vi "Шифр Хилла.vi"() -> ()   [LabVIEW 2016]
uses:
  <vilib>/Analysis/Matrix/Datatypes/RealMatrix.ctl
  <vilib>/silver_ctls/ArrayMatrixCluster/Real Matrix NI_Silver.ctl
  Dll_Hill/Dll_Hill/Dll_Hill/bin/Debug/Dll_Hill.dll
  <vilib>/Analysis/baseanly.llb/Real Determinant.vi
  <vilib>/Analysis/baseanly.llb/Vector x A.vi
  <vilib>/Analysis/baseanly.llb/Real A x B.vi
  <vilib>/Analysis/Matrix/Numeric/Conversions/Array To Matrix - RA.vi
  <vilib>/Analysis/Matrix/Numeric/Conversions/Matrix To Array - RM.vi
  <vilib>/Analysis/NI_AALBase.lvlib
  <vilib>/Analysis/Matrix/NI_Matrix.lvlib
panel:
  in  "Главное меню":T1(tab)
  in  "Укажите путь к входному алфавиту":path
  in  "Путь к алфавиту":bool
  in  "Выход":bool
  out "Входной алфавит":string
  out "index":i32[](array[numeric])
  in  "Введите входное слово":string
  in  "Введите ключ":string
  in  "Получение ключа и входного сообщения":bool
  out "Полученный ключ":string
  out "Матрица ключа":T2
  in  "Строки матрицы ключа":i32
  in  "Столбцы матрицы ключа":i32
  out "Полученное входное слово":string
  out "Вектор входного слова":i32[](array[numeric])
  in  "дл.исх.сообщ.":i32
  out "Зашифрованный вектор_2":string[][](table)
  in  "Шифрование":bool
  out "Матрица ключа * Матрицу вх. сообщ.":dbl[](array[numeric]) format="%.2f"
  out "Зашифрованный вектор":dbl[](array[numeric])
  out "Определитель матрицы ключа":i32
  in  "Пользовательский пример.\nУкажите путь к файлу  в Подменю\n\"Пользовательский пример\"\nперед нажатием на кнопку - \n\"Пользовательский пример\"":bool
  in  "Расшифрование":bool
  in  "Выход в главное меню":bool
  in  "Подменю":T3(tab)
  out "Зашифрованное сообщение_2":string[][](table)
  in  "Зашифрованное сообщение":string
  in  "Закодированный ключ_р":T4
  in  "Укажите путь к  алфавиту дешифрования":path
  out "Зашифрованный ключ_р_2":string[][](table)
  out "Исходное сообщение":dbl[](array[numeric])
  out "Исходное сообщение":string
  in  "дл.исх.сообщ.":i32
  out "y":i64[](array[numeric])
  out "x":i64[](array[numeric])
  out "d":i64[](array[numeric])
  out "pow":i32
  out "минор":i32
  out "invert_det":i64
  out "опред  минора":T2
  out "Проверка":T2
  out "обратная по модулю к матрице ключа":T2
  out "Матрица миноров":T2
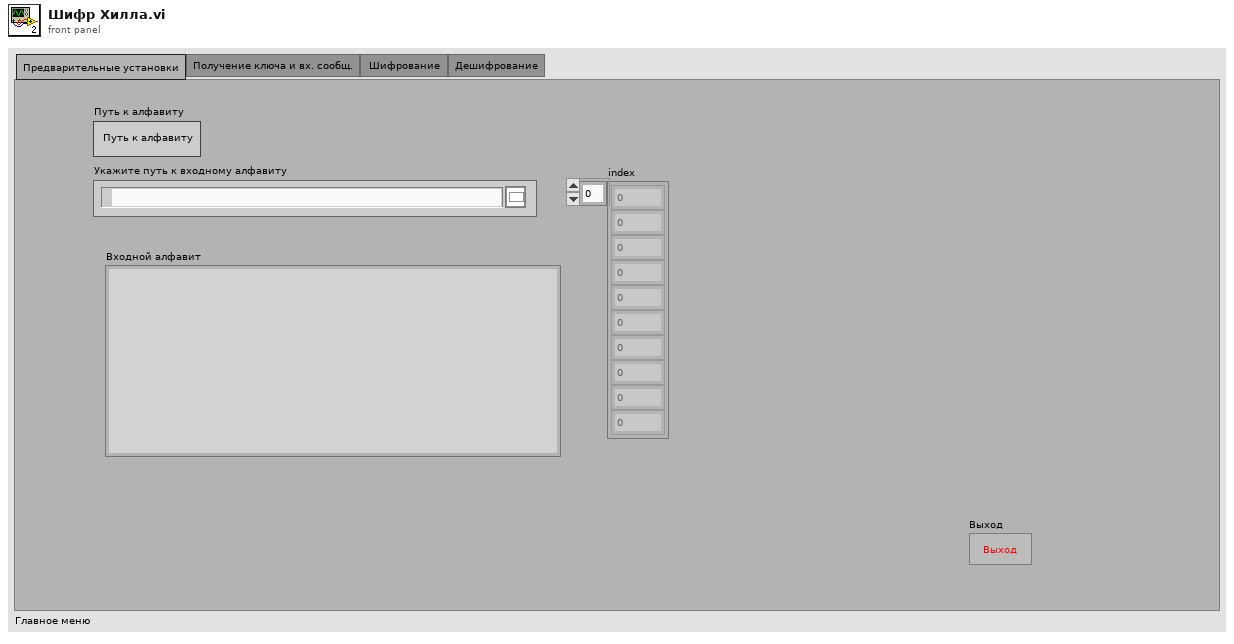
[diagram p1: front panel]
types:
  T1 = enum32{"Предварительные установки", "Получение ключа и вх. сообщ.", "Шифрование ", "Дешифрование"}
  T2 = typedef "NI_Matrix.lvlib/RealMatrix.ctl" = dbl[][]
  T3 = enum32{"Пользовательский пример", "Пользовательский пример шаг_2"}
  T4 = typedef "Real Matrix NI_Silver.ctl" = dbl[][]
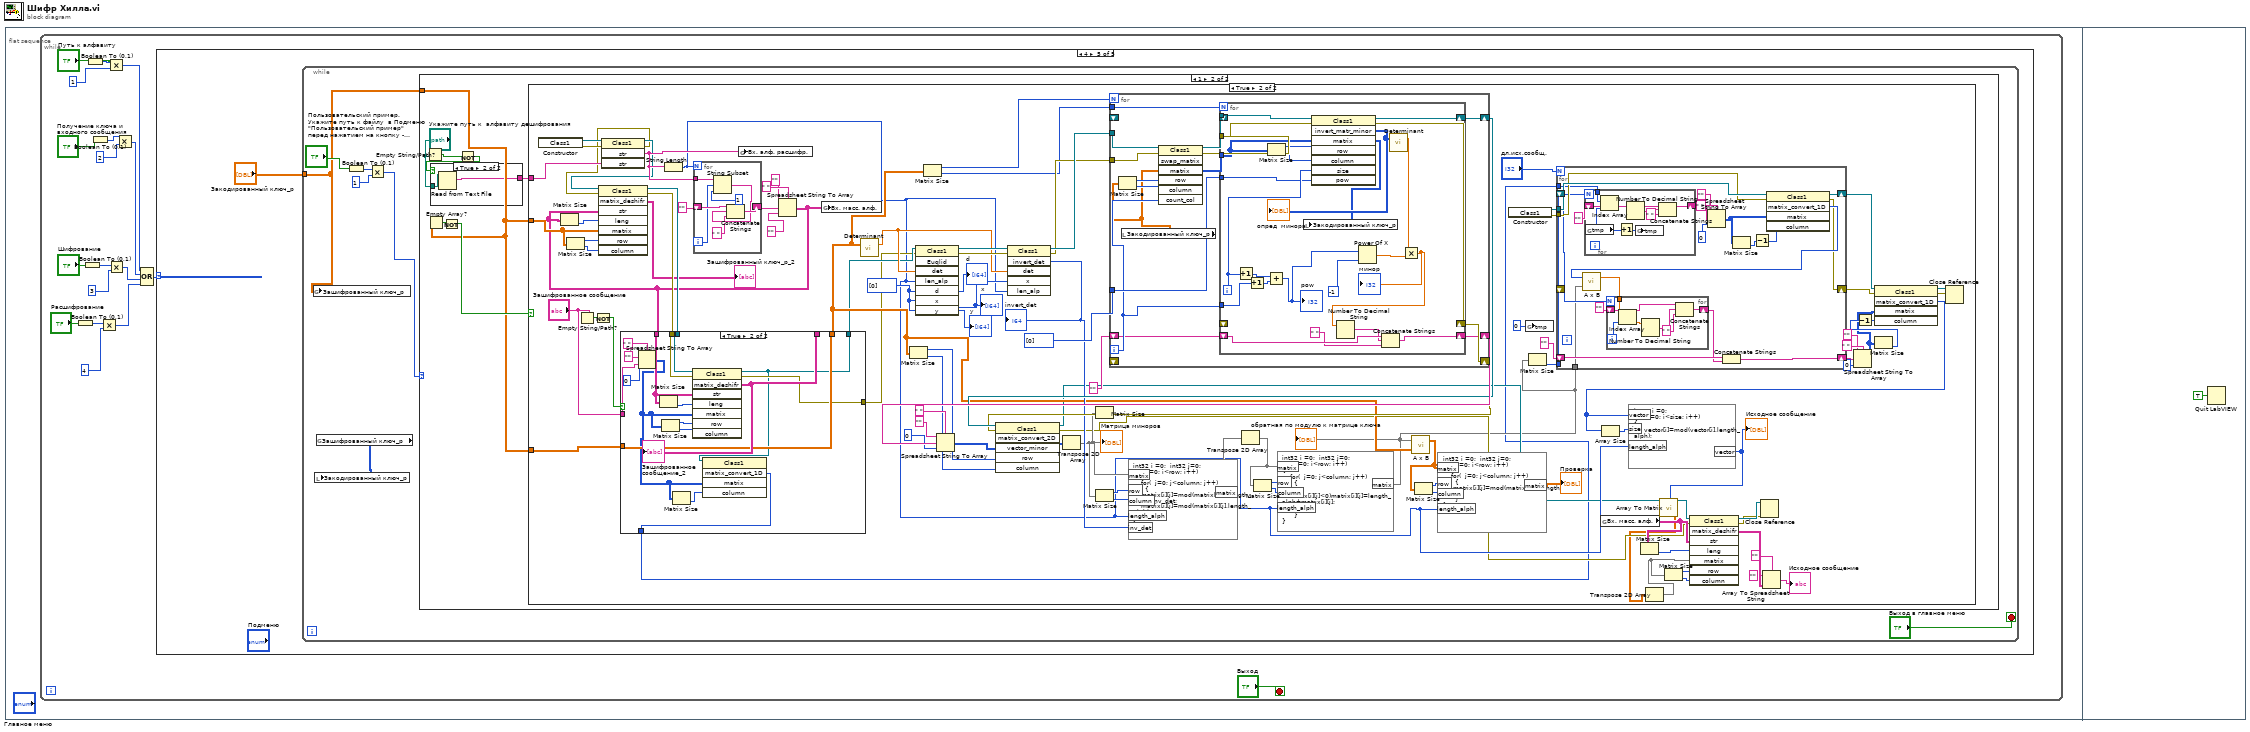
[diagram p0: block diagram]
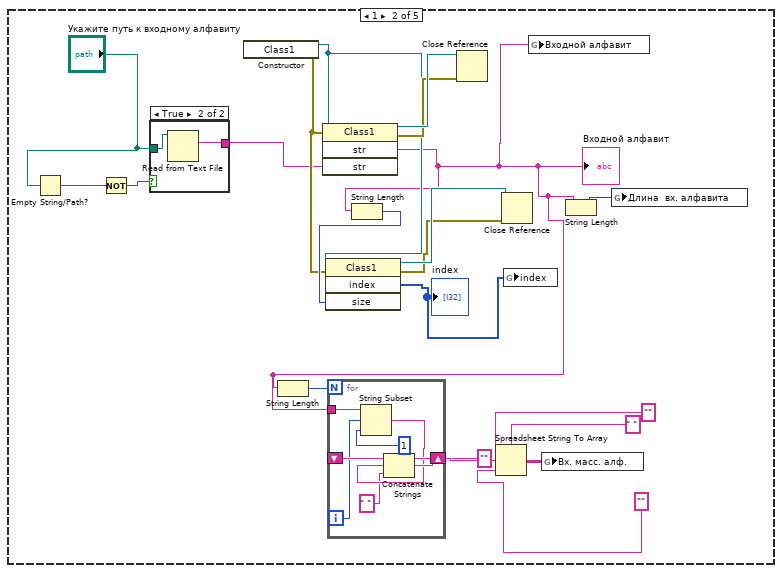
[diagram p3: hidden frame]
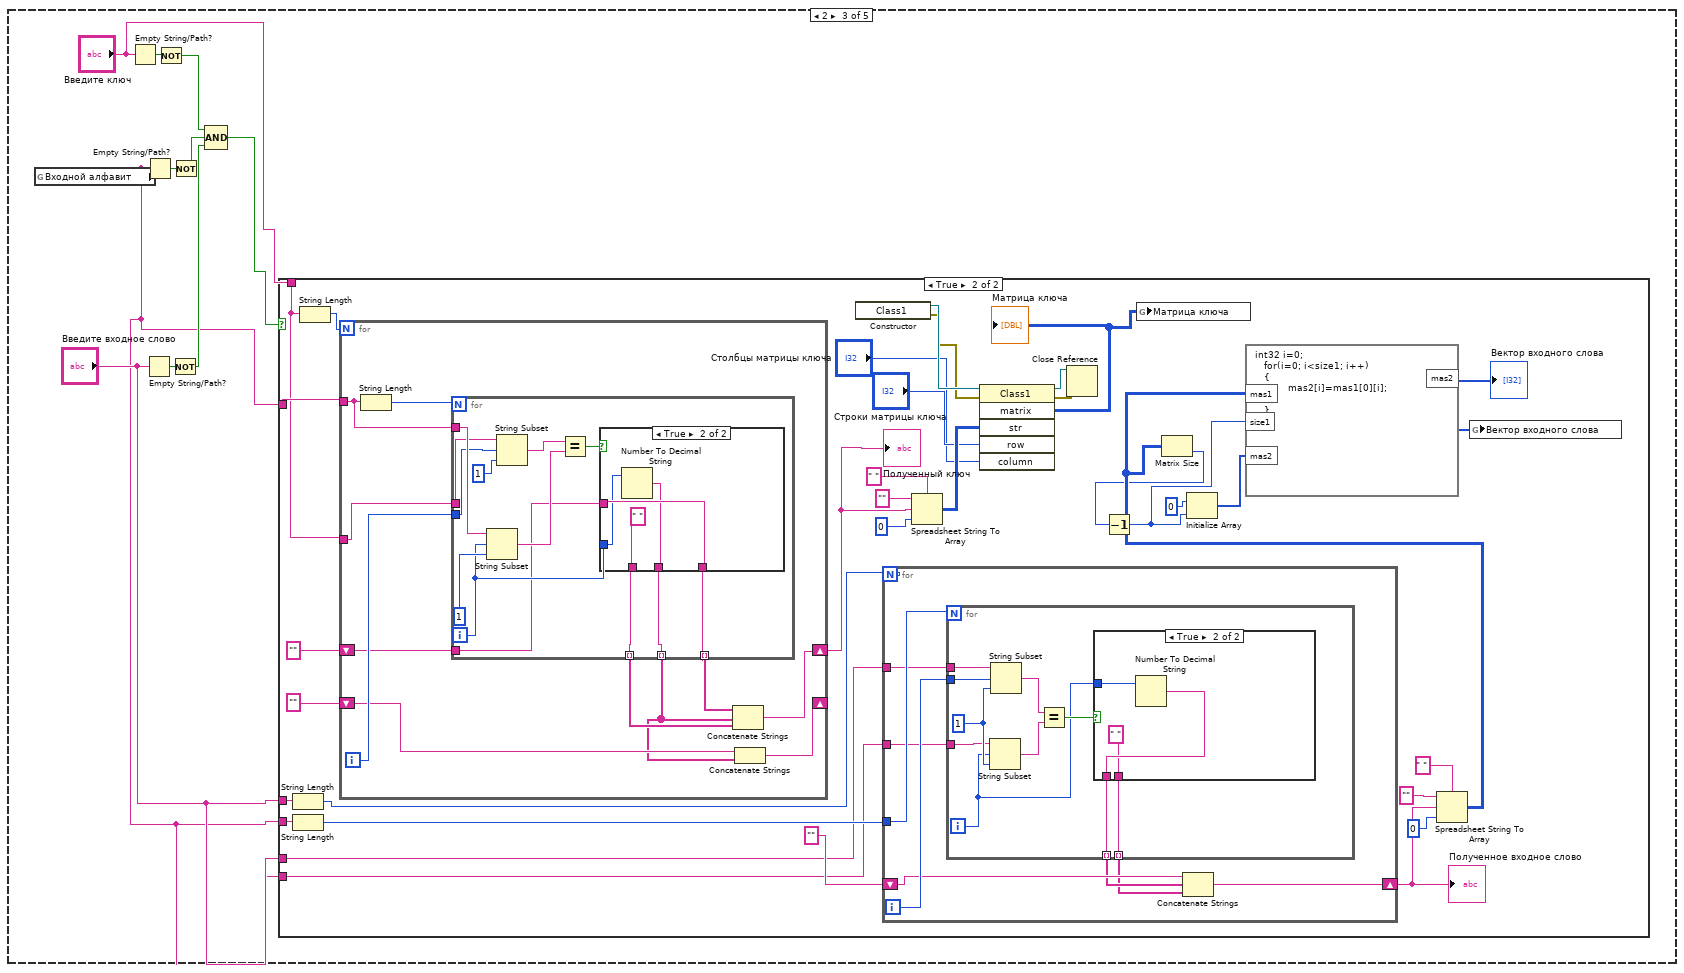
[diagram p5: hidden frame]
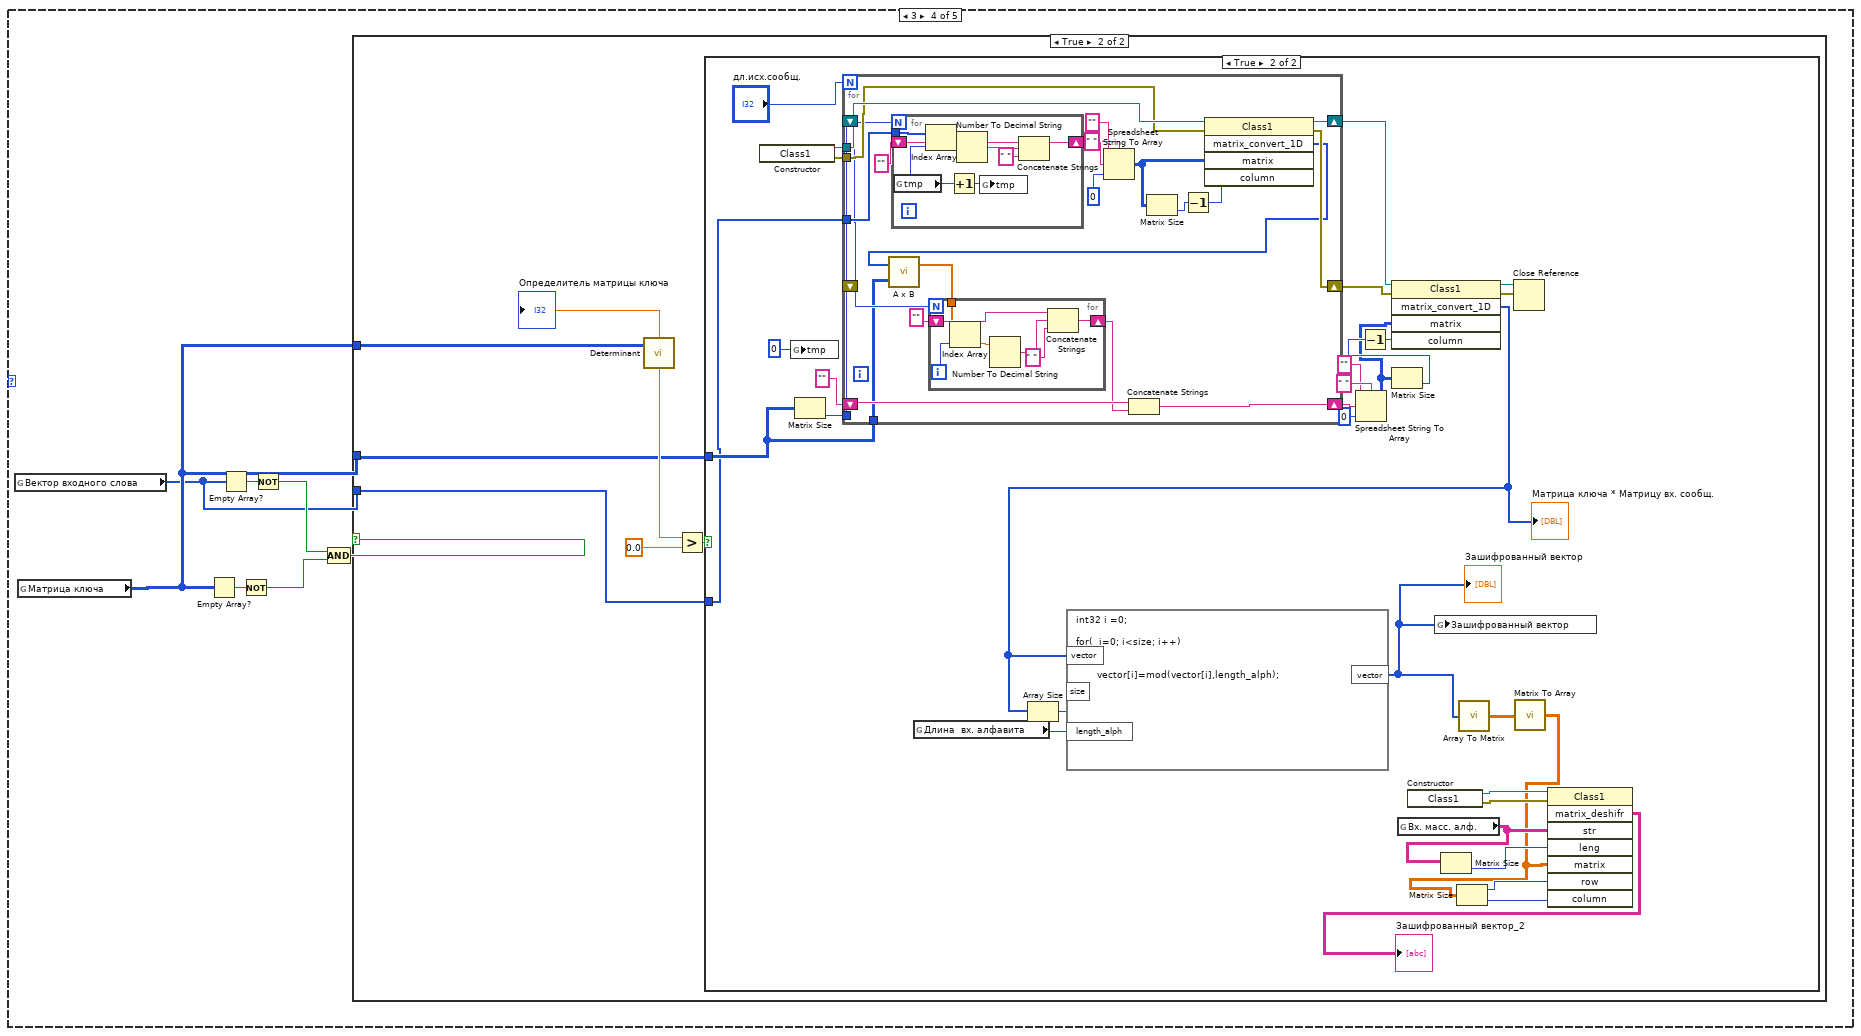
[diagram p9: hidden frame]
diagram:
  n1 = flat-sequence {
    frame #0 {
      n2 = while {
        stop <- "Выход" stop-if-true
        n3 = Boolean To (0,1)(Boolean="Расшифрование") -> (0, 1=w2:i16)
        n4 = Boolean To (0,1)(Boolean="Шифрование") -> (0, 1=w6:i16)
        n5 = Boolean To (0,1)(Boolean="Путь к алфавиту") -> (0, 1=w16:i16)
        n6 = Boolean To (0,1)(Boolean="Получение ключа и входного сообщения") -> (0, 1=w13:i16)
        n7 = Multiply(x=w2, y=4) -> (x*y=w1:i32)
        n8 = Multiply(x=w16, y=1) -> (x*y=w10:i32)
        n9 = Multiply(x=w6, y=3) -> (x*y=w5:i32)
        n10 = Multiply(x=w13, y=2) -> (x*y=w9:i32)
        n11 = Compound Arithmetic op=OR(w10, w9, w5, w1) -> (w15:i32)
        n12 = case shown="4" w15 {
          frame 0, Default {
          }
          frame 1 {
            n13 = Empty String/Path?(string/path="Укажите путь к входному алфавиту") -> (empty?=w31:bool)
            n14 = Not(x=w31) -> (.not. x?=w30:bool)
            n15 = case shown="True" w30 {
              tunnel: "Укажите путь к входному алфавиту" -> [_ w48]
              tunnel: [_ w47] -> w28
              frame False {
              }
              frame True {
                n16 = Read from Text File(file (use dialog)=w48) -> (text=w47:string)  [unwired: 3 in, 3 out]
              }
            }
            n17 = constructor class="Class1"() -> (reference out=w37:refnum<k24>, error out=w35:errorcluster)  [unwired: 3 in, 1 out]
            n18 = invoke class="Class1" method="str"(reference=w37, error in=w35, "str"=w28) -> (reference out=w39:refnum<k24>, error out=w38:errorcluster, "str"=w19:string)  [unwired: 1 in, 1 out]
            "Входной алфавит" <- w19
            n19 = String Length(string=w19) -> (length=w21:i32)
            n20 = for {
              N: w21 -> [_]
              shift-right: [w46] -> w23
              shift-left: "" -> [w45]
              tunnel: w19 -> [w40]
              i -> [w43]
              n21 = String Subset(string=w40, offset (0)=w43, length (rest)=1 ("length (rest)")) -> (substring=w42:string)
              n22 = Concatenate Strings(w45, w42, " ") -> (w46:string)
            }
            n23 = String Length(string=w19) -> (length=w36:i32)
            n24 = invoke class="Class1" method="index"(reference=w37, error in=w35, "size"=w36) -> (reference out=w34:refnum<k24>, error out=w33:errorcluster, "index"=w32:i32[])  [unwired: 1 in, 1 out]
            "index" <- w32
            n25 = Close Reference(reference=w39, error in (no error)=w38) -> ()  [unwired: 1 out]
            n26 = Spreadsheet String To Array(delimiter (Tab)=" ", format string="", spreadsheet string=w23, array type (2D Dbl)="") -> (array=w20:string[][])
            n27 = Close Reference(reference=w34, error in (no error)=w33) -> ()  [unwired: 1 out]
            n28 = global write "Global 1.vi" "index"(w32) -> ()
            n29 = global write "Global 1.vi" "Входной алфавит"(w19) -> ()
            n30 = global write "Global 1.vi" "Вх. масс. алф."(w20) -> ()
            n31 = String Length(string=w19) -> (length=w27:i32)
            n32 = global write "Global 1.vi" "Длина  вх. алфавита"(w27) -> ()
          }
          frame 2 {
            n33 = global read "Global 1.vi" "Входной алфавит"() -> (w49:string)
            n34 = Empty String/Path?(string/path="Введите ключ") -> (empty?=w58:bool)
            n35 = Empty String/Path?(string/path="Введите входное слово") -> (empty?=w52:bool)
            n36 = Empty String/Path?(string/path=w49) -> (empty?=w57:bool)
            n37 = Not(x=w58) -> (.not. x?=w55:bool)
            n38 = Not(x=w52) -> (.not. x?=w51:bool)
            n39 = Not(x=w57) -> (.not. x?=w54:bool)
            n40 = Compound Arithmetic op=AND(w55, w54, w51) -> (w53:bool)
            n41 = case shown="True" w53 {
              tunnel: "Введите ключ" -> [_ w90]
              tunnel: w49 -> [_ w91]
              tunnel: "Введите входное слово" -> [_ w76]
              tunnel: w49 -> [_ w74]
              tunnel: "Введите входное слово" -> [_ w71]
              tunnel: w49 -> [_ w70]
              frame False {
              }
              frame True {
                n42 = String Length(string=w76) -> (length=w75:i32)
                n43 = String Length(string=w74) -> (length=w73:i32)
                n44 = String Length(string=w90) -> (length=w92:i32)
                n45 = for {
                  N: w92 -> [_]
                  tunnel: w91 -> [w123]
                  tunnel: w90 -> [w122]
                  shift-right: [w118] -> w82
                  shift-left: "" -> [w120]
                  shift-right: [w114] -> _
                  shift-left: "" -> [w116]
                  i -> [w121]
                  n46 = String Length(string=w123) -> (length=w124:i32)
                  n47 = for {
                    N: w124 -> [_]
                    tunnel: w123 -> [w136]
                    tunnel: w122 -> [w134]
                    tunnel: w121 -> [w132]
                    tunnel: w120 -> [w128]
                    tunnel: [w127] -> w119 mode=indexing
                    tunnel: [w126] -> w115 mode=indexing
                    tunnel: [w125] -> w117 mode=indexing
                    i -> [w130]
                    n48 = String Subset(string=w136, offset (0)=w130, length (rest)=1 ("length (rest)")) -> (substring=w129:string)
                    n49 = String Subset(string=w134, offset (0)=w132, length (rest)=1 ("length (rest)")) -> (substring=w131:string)
                    n50 = Equal?(x=w131, y=w129) -> (x = y?=w135:bool)
                    n51 = case shown="True" w135 {
                      tunnel: w130 -> [_ w140]
                      tunnel: w128 -> [_ w141]
                      tunnel: [_ w141] -> w127
                      tunnel: [_ w139] -> w126
                      tunnel: [_ " "] -> w125
                      frame False {
                      }
                      frame True {
                        n52 = Number To Decimal String(number=w140) -> (decimal integer string=w139:string)  [unwired: 1 in]
                      }
                    }
                  }
                  n53 = Concatenate Strings(w119, w115, w117) -> (w118:string)
                  n54 = Concatenate Strings(w116, w115) -> (w114:string)
                }
                "Полученный ключ" <- w82
                n55 = constructor class="Class1"() -> (reference out=w88:refnum<k24>, error out=w87:errorcluster)  [unwired: 3 in, 1 out]
                n56 = for {
                  N: w75 -> [_]
                  tunnel: w73 -> [w100]
                  shift-right: [w93] -> w69
                  shift-left: "" -> [w96]
                  tunnel: w71 -> [w98]
                  tunnel: w70 -> [w97]
                  i -> [w99]
                  n57 = for {
                    N: w100 -> [_]
                    tunnel: w99 -> [w110]
                    tunnel: w98 -> [w109]
                    tunnel: w97 -> [w107]
                    tunnel: [w102] -> w95 mode=indexing
                    tunnel: [w101] -> w94 mode=indexing
                    i -> [w103]
                    w108 = 1 ("length (rest)")
                    n58 = String Subset(string=w107, offset (0)=w103, length (rest)=w108) -> (substring=w105:string)
                    n59 = String Subset(string=w109, offset (0)=w110, length (rest)=w108) -> (substring=w106:string)
                    n60 = Equal?(x=w106, y=w105) -> (x = y?=w104:bool)
                    n61 = case shown="True" w104 {
                      tunnel: w103 -> [_ w113]
                      tunnel: [_ w112] -> w102
                      tunnel: [_ " "] -> w101
                      frame False {
                      }
                      frame True {
                        n62 = Number To Decimal String(number=w113) -> (decimal integer string=w112:string)  [unwired: 1 in]
                      }
                    }
                  }
                  n63 = Concatenate Strings(w96, w95, w94) -> (w93:string)
                }
                "Полученное входное слово" <- w69
                n64 = Spreadsheet String To Array(delimiter (Tab)=" ", format string="", spreadsheet string=w82, array type (2D Dbl)=0) -> (array=w79:i32[][])
                n65 = invoke class="Class1" method="matrix"(reference=w88, error in=w87, "str"=w79, "row"="Строки матрицы ключа", "column"="Столбцы матрицы ключа") -> (reference out=w85:refnum<k24>, error out=w86:errorcluster, "matrix"=w59:i32[][])  [unwired: 1 in, 3 out]
                "Матрица ключа" <- w59
                n66 = Close Reference(reference=w85, error in (no error)=w86) -> ()  [unwired: 1 out]
                n67 = global write "Global 1.vi" "Матрица ключа"(w59) -> ()
                n68 = Spreadsheet String To Array(delimiter (Tab)=" ", format string="", spreadsheet string=w69, array type (2D Dbl)=0) -> (array=w65:i32[][])
                n69 = Matrix Size(0:w65) -> (2:w62:i32)  [unwired: 1 out]
                n70 = Decrement(x=w62) -> (x-1=w61:i32)
                n71 = Initialize Array(0 ("element"), w61) -> (w63:i32[])
                n72 = formula code="int32 i=0;\n   for(i=0; i<size1; i++)\n   {\n           mas2[i]=mas1[0][i];\n   \n   }"("mas1"=w65, "size1"=w61, "mas2"=w63) -> ("mas2"=w60:i32[])
                "Вектор входного слова" <- w60
                n73 = global write "Global 1.vi" "Вектор входного слова"(w60) -> ()
              }
            }
          }
          frame 3 {
            n74 = global read "Global 1.vi" "Вектор входного слова"() -> (w142:i32[])
            n75 = global read "Global 1.vi" "Матрица ключа"() -> (w143:i32[][])
            n76 = Empty Array?(array=w143) -> (empty?=w148:bool)
            n77 = Empty Array?(array=w142) -> (empty?=w147:bool)
            n78 = Not(x=w148) -> (.not. x?=w145:bool)
            n79 = Not(x=w147) -> (.not. x?=w146:bool)
            n80 = Compound Arithmetic op=AND(w146, w145) -> (w144:bool)
            n81 = case shown="True" w144 {
              tunnel: w143 -> [_ w154]
              tunnel: w143 -> [_ w150]
              tunnel: w142 -> [_ w149]
              frame False {
              }
              frame True {
                n82 = call-poly <vilib>:"Determinant.vi"("Input Matrix"=w154) -> ("determinant"=w153:dbl)  [unwired: 1 in, 1 out]
                "Определитель матрицы ключа" <- w153
                n83 = Greater?(x=w153, y=0.0) -> (0:w151:bool)
                n84 = case shown="True" w151 {
                  tunnel: w150 -> [_ w174]
                  tunnel: w149 -> [_ w171]
                  frame False {
                  }
                  frame True {
                    n85 = constructor class="Class1"() -> (reference out=w173:refnum<k24>, error out=w169:errorcluster)  [unwired: 3 in, 1 out]
                    n86 = global write "Global 1.vi" "tmp"(0 ("Numeric Control")) -> ()
                    n87 = Matrix Size(0:w174) -> (2:w175:i32)  [unwired: 1 out]
                    n88 = for {
                      N: "дл.исх.сообщ." -> [_]
                      tunnel: w175 -> [w192]
                      tunnel: w174 -> [w188]
                      tunnel: w171 -> [w206]
                      tunnel: w173 -> [w201]
                      tunnel: w169 -> [w199]
                      shift-right: [w197] -> w164
                      shift-left: "" -> [w198]
                      shift-right: [w190] -> w159
                      shift-left: _ -> [_]
                      shift-right: [w189] -> w158
                      shift-left: _ -> [_]
                      n89 = for {
                        N: w192 -> [_]
                        shift-right: [w215] -> w205
                        shift-left: "" -> [w219]
                        tunnel: w206 -> [w220]
                        n90 = global read "Global 1.vi" "tmp"() -> (w221:i32)
                        n91 = Index Array(array=w220, index=w221) -> (element=w217:i32)
                        n92 = Increment(x=w221) -> (x+1=w222:i32)
                        n93 = Number To Decimal String(number=w217) -> (decimal integer string=w218:string)  [unwired: 1 in]
                        n94 = global write "Global 1.vi" "tmp"(w222) -> ()
                        n95 = Concatenate Strings(w219, w218, " ") -> (w215:string)
                      }
                      n96 = Spreadsheet String To Array(delimiter (Tab)=" ", format string="", spreadsheet string=w205, array type (2D Dbl)=0) -> (array=w194:i32[][])
                      n97 = Matrix Size(0:w194) -> (2:w195:i32)  [unwired: 1 out]
                      n98 = Decrement(x=w195) -> (x-1=w196:i32)
                      n99 = invoke class="Class1" method="matrix_convert_1D"(reference=w201, error in=w199, "matrix"=w194, "column"=w196) -> (reference out=w190:refnum<k24>, error out=w189:errorcluster, "matrix_convert_1D"=w187:i32[])  [unwired: 1 in, 2 out]
                      n100 = call-poly <vilib>:"A x B.vi"("Matrix A"=w188, "Vector V'"=w187) -> ("V' x A"=w193:dbl[])  [unwired: 1 out]
                      n101 = for {
                        N: w192 -> [_]
                        shift-right: [w211] -> w191
                        shift-left: "" -> [w214]
                        tunnel: w193 -> [w209]
                        i -> [w210]
                        n102 = Index Array(array=w209, index=w210) -> (element=w208:dbl)
                        n103 = Number To Decimal String(number=w208) -> (decimal integer string=w213:string)  [unwired: 1 in]
                        n104 = Concatenate Strings(w214, w213, " ") -> (w211:string)
                      }
                      n105 = Concatenate Strings(w198, w191) -> (w197:string)
                    }
                    n106 = global read "Global 1.vi" "Длина  вх. алфавита"() -> (w184:i32)
                    n107 = Spreadsheet String To Array(delimiter (Tab)=" ", format string="", spreadsheet string=w164, array type (2D Dbl)=0) -> (array=w161:i32[][])
                    n108 = Matrix Size(0:w161) -> (2:w163:i32)  [unwired: 1 out]
                    n109 = Decrement(x=w163) -> (x-1=w162:i32)
                    n110 = invoke class="Class1" method="matrix_convert_1D"(reference=w159, error in=w158, "matrix"=w161, "column"=w162) -> (reference out=w157:refnum<k24>, error out=w156:errorcluster, "matrix_convert_1D"=w155:i32[])  [unwired: 1 in, 2 out]
                    "Матрица ключа * Матрицу вх. сообщ." <- w155
                    n111 = Array Size(array=w155) -> (size(s)=w160:i32)
                    n112 = formula code="int32 i =0;\n\nfor(  i=0; i<size; i++)\n{\n      \n       vector[i]=mod(vector[i],length_alph);\n\n}"("vector"=w155, "size"=w160, "length_alph"=w184) -> ("vector"=w172:i32[])
                    "Зашифрованный вектор" <- w172
                    n113 = global read "Global 1.vi" "Вх. масс. алф."() -> (w183:string[][])
                    n114 = constructor class="Class1"() -> (reference out=w186:refnum<k24>, error out=w185:errorcluster)  [unwired: 3 in, 1 out]
                    n115 = global write "Global 1.vi" "Зашифрованный вектор"(w172) -> ()
                    n116 = Matrix Size(0:w183) -> (2:w182:i32)  [unwired: 1 out]
                    n117 = call-poly <vilib>:"Array To Matrix.vi"("Real 1D Array"=w172) -> ("Real Matrix (Column Vector)"=w180:T2)
                    n118 = Close Reference(reference=w157, error in (no error)=w156) -> ()  [unwired: 1 out]
                    n119 = call-poly <vilib>:"Matrix To Array.vi"("Real Matrix"=w180) -> ("Real 2D Array"=w177:dbl[][])
                    n120 = Matrix Size(0:w177) -> (1:w179:i32, 2:w178:i32)
                    n121 = invoke class="Class1" method="matrix_deshifr"(reference=w186, error in=w185, "str"=w183, "leng"=w182, "matrix"=w177, "row"=w179, "column"=w178) -> ("matrix_deshifr"=→"Зашифрованный вектор_2":string[][])  [unwired: 1 in, 7 out]
                  }
                }
              }
            }
          }
          frame 4 {
            n122 = while {
              tunnel: "Закодированный ключ_р" -> [w225]
              stop <- "Выход в главное меню" stop-if-true
              n123 = global write "Global 1.vi" "Зашифрованный ключ_р"(w225) -> ()
              n124 = global read "Global 1.vi" "Зашифрованный ключ_р"() -> (w224:i32[][])
              n125 = local write "Закодированный ключ_р"(w224) -> ()
              n126 = Boolean To (0,1)(Boolean="Пользовательский пример.\nУкажите путь к файлу  в Подменю\n\"Пользовательский пример\"\nперед нажатием на кнопку - \n\"Пользовательский пример\"") -> (0, 1=w229:i16)
              n127 = Multiply(x=w229, y=1) -> (x*y=w226:i32)
              n128 = case shown="1" w226 {
                tunnel: w225 -> [_ w231]
                frame 0, Default {
                }
                frame 1 {
                  n129 = Empty String/Path?(string/path="Укажите путь к  алфавиту дешифрования") -> (empty?=w237:bool)
                  n130 = Empty Array?(array=w231) -> (empty?=w234:bool)
                  n131 = Not(x=w234) -> (.not. x?=w233:bool)
                  n132 = Not(x=w237) -> (.not. x?=w236:bool)
                  n133 = case shown="True" w236 {
                    tunnel: "Укажите путь к  алфавиту дешифрования" -> [_ w435]
                    tunnel: [_ w434] -> w232
                    frame False {
                    }
                    frame True {
                      n134 = Read from Text File(file (use dialog)=w435) -> (text=w434:string)  [unwired: 3 in, 3 out]
                    }
                  }
                  n135 = case shown="True" w233 {
                    tunnel: w232 -> [_ w335]
                    tunnel: w231 -> [_ w321]
                    tunnel: w231 -> [_ w314]
                    frame False {
                    }
                    frame True {
                      w312 = i64[] [0] ("d")
                      n136 = constructor class="Class1"() -> (reference out=w330:refnum<k24>, error out=w329:errorcluster)  [unwired: 3 in, 1 out]
                      n137 = Matrix Size(0:w321) -> (1:w323:i32, 2:w322:i32)
                      n138 = Empty String/Path?(string/path="Зашифрованное сообщение") -> (empty?=w320:bool)
                      n139 = Not(x=w320) -> (.not. x?=w319:bool)
                      n140 = invoke class="Class1" method="str"(reference=w330, error in=w329, "str"=w335) -> (reference out=w328:refnum<k24>, error out=w327:errorcluster, "str"=w333:string)  [unwired: 1 in, 1 out]
                      n141 = String Length(string=w333) -> (length=w274:i32)
                      n142 = for {
                        N: w274 -> [_]
                        shift-right: [w433] -> w326
                        shift-left: "" -> [w432]
                        tunnel: w333 -> [w431]
                        i -> [w429]
                        n143 = String Subset(string=w431, offset (0)=w429, length (rest)=1 ("length (rest)")) -> (substring=w428:string)
                        n144 = Concatenate Strings(w432, w428, " ") -> (w433:string)
                      }
                      n145 = global write "Global 1.vi" "Вх. алф. расшифр."(w333) -> ()
                      n146 = Spreadsheet String To Array(delimiter (Tab)=" ", format string="", spreadsheet string=w326, array type (2D Dbl)="") -> (array=w313:string[][])
                      n147 = Matrix Size(0:w313) -> (2:w324:i32)  [unwired: 1 out]
                      n148 = invoke class="Class1" method="matrix_deshifr"(reference=w328, error in=w327, "str"=w313, "leng"=w324, "matrix"=w321, "row"=w323, "column"=w322) -> (reference out=w317:refnum<k24>, error out=w316:errorcluster, "matrix_deshifr"=→"Зашифрованный ключ_р_2":string[][])  [unwired: 1 in, 5 out]
                      n149 = case shown="True" w319 {
                        tunnel: "Зашифрованное сообщение" -> [_ w423]
                        tunnel: w317 -> [_ w422]
                        tunnel: w316 -> [_ w421]
                        tunnel: w313 -> [_ w420]
                        tunnel: [_ w417] -> _
                        tunnel: [_ w415] -> w282
                        tunnel: w314 -> [_ w415]
                        tunnel: [_ w411] -> w278
                        tunnel: [_ w414] -> w277
                        tunnel: [_ w410] -> w238
                        frame False {
                        }
                        frame True {
                          n150 = Spreadsheet String To Array(delimiter (Tab)=" ", format string="", spreadsheet string=w423, array type (2D Dbl)=0) -> (array=w413:i32[][])
                          n151 = Matrix Size(0:w420) -> (2:w419:i32)  [unwired: 1 out]
                          n152 = Matrix Size(0:w413) -> (1:w416:i32, 2:w418:i32)
                          n153 = Matrix Size(0:w413) -> (2:w412:i32)  [unwired: 1 out]
                          n154 = invoke class="Class1" method="matrix_deshifr"(reference=w422, error in=w421, "str"=w420, "leng"=w419, "matrix"=w413, "row"=w416, "column"=w418) -> (reference out=w411:refnum<k24>, error out=w414:errorcluster, "matrix_deshifr"=w417:string[][])  [unwired: 1 in, 5 out]
                          "Зашифрованное сообщение_2" <- w417
                          n155 = invoke class="Class1" method="matrix_convert_1D"(reference=w411, "matrix"=w413, "column"=w412) -> ("matrix_convert_1D"=w410:i32[])  [unwired: 2 in, 4 out]
                        }
                      }
                      n156 = global write "Global 1.vi" "Вх. масс. алф."(w313) -> ()
                      n157 = call-poly <vilib>:"Determinant.vi"("Input Matrix"=w282) -> ("determinant"=w307:dbl)  [unwired: 1 in, 1 out]
                      n158 = Matrix Size(0:w282) -> (1:w292:i32, 2:w291:i32)
                      n159 = invoke class="Class1" method="Euqlid"(reference=w278, error in=w277, "det"=w307, "len_alp"=w274, "d"=w312, "x"=w312, "y"=w312) -> (reference out=w309:refnum<k24>, error out=w308:errorcluster, "d"=→"d":i64[], "x"=w306:i64[], "y"=→"y":i64[])  [unwired: 1 in, 3 out]
                      "x" <- w306
                      n160 = Matrix Size(0:w282) -> (1:w297:i32, 2:w296:i32)
                      n161 = invoke class="Class1" method="invert_det"(reference=w309, error in=w308, "det"=w307, "x"=w306, "len_alp"=w274) -> (reference out=w305:refnum<k24>, error out=w303:errorcluster, "invert_det"=w287:i64)  [unwired: 1 in, 3 out]
                      "invert_det" <- w287
                      n162 = for {
                        N: w297 -> [_]
                        tunnel: w305 -> [w384]
                        tunnel: i32[] [0] ("pow") -> [w380]
                        tunnel: w303 -> [w383]
                        shift-right: [w372] -> w301
                        shift-left: "" -> [w373]
                        tunnel: w296 -> [w376]
                        shift-right: [w375] -> w295
                        shift-left: _ -> [_]
                        shift-right: [w374] -> w294
                        shift-left: _ -> [_]
                        i -> [w379]
                        n163 = local read "Закодированный ключ_р"() -> (w377:T4)
                        n164 = Matrix Size(0:w377) -> (1:w385:i32, 2:w386:i32)
                        n165 = invoke class="Class1" method="swap_matrix"(reference=w384, error in=w383, "matrix"=w377, "row"=w385, "column"=w386, "count_col"=w379) -> (reference out=w382:refnum<k24>, error out=w381:errorcluster, "matrix"=w378:i32[][])  [unwired: 1 in, 4 out]
                        n166 = for {
                          N: w376 -> [_]
                          tunnel: w382 -> [w403]
                          tunnel: w381 -> [w402]
                          tunnel: w380 -> [w399]
                          tunnel: w379 -> [w397]
                          tunnel: w378 -> [w395]
                          shift-right: [w392] -> w375
                          shift-left: _ -> [_]
                          shift-right: [w391] -> w374
                          shift-left: _ -> [_]
                          shift-right: [w387] -> w372
                          shift-left: w373 -> [w390]
                          i -> [w404]
                          n167 = Increment(x=w404) -> (x+1=w409:i32)
                          n168 = Increment(x=w397) -> (x+1=w408:i32)
                          n169 = Matrix Size(0:w395) -> (1:w401:i32, 2:w400:i32)
                          n170 = Add(x=w409, y=w408) -> (x+y=w406:i32)
                          "pow" <- w406
                          n171 = invoke class="Class1" method="invert_matr_minor"(reference=w403, error in=w402, "matrix"=w395, "row"=w401, "column"=w400, "size"=w404, "pow"=w399) -> (reference out=w392:refnum<k24>, error out=w391:errorcluster, "invert_matr_minor"=w398:i32[][], "matrix"=w396:i32[][])  [unwired: 1 in, 4 out]
                          "опред  минора" <- w398
                          n172 = local write "Закодированный ключ_р"(w396) -> ()
                          n173 = Power Of X(1:-1 ("x"), 2:w406) -> (0:w405:dbl)
                          n174 = call-poly <vilib>:"Determinant.vi"("Input Matrix"=w398) -> ("determinant"=w394:dbl)  [unwired: 1 in, 1 out]
                          n175 = Multiply(x=w394, y=w405) -> (x*y=w393:dbl)
                          "минор" <- w393
                          n176 = Number To Decimal String(number=w393) -> (decimal integer string=w389:string)  [unwired: 1 in]
                          n177 = Concatenate Strings(w390, w389, " ") -> (w387:string)
                        }
                      }
                      n178 = Spreadsheet String To Array(delimiter (Tab)=" ", format string="", spreadsheet string=w301, array type (2D Dbl)=0) -> (array=w293:i32[][])
                      n179 = invoke class="Class1" method="matrix_convert_2D"(reference=w295, error in=w294, "vector_minor"=w293, "row"=w292, "column"=w291) -> (reference out=w267:refnum<k24>, error out=w266:errorcluster, "matrix_convert_2D"=w290:i32[][])  [unwired: 1 in, 3 out]
                      n180 = Transpose 2D Array(2D array=w290) -> (transposed array=w275:i32[][])
                      "Матрица миноров" <- w275
                      n181 = Matrix Size(0:w275) -> (1:w289:i32, 2:w288:i32)
                      n182 = Matrix Size(0:w275) -> ()  [unwired: 2 out]
                      n183 = formula code="int32 i =0;  int32 j=0;\nfor(  i=0; i<row; i++)\n{\n    for(  j=0; j<column; j++)\n      {\n    matrix[i][j]=mod(matrix[i][j],length_alph)*inv_det;\n    matrix[i][j]=mod(matrix[i][j],length_alph);\n      }\n}"("matrix"=w275, "length_alph"=w274, "column"=w288, "row"=w289, "inv_det"=w287) -> ("matrix"=w286:i32[][])
                      n184 = Transpose 2D Array(2D array=w286) -> (transposed array=w285:i32[][])
                      n185 = Matrix Size(0:w285) -> (1:w284:i32, 2:w283:i32)
                      n186 = formula code="int32 i =0;  int32 j=0;\nfor(  i=0; i<row; i++)\n{\n    for(  j=0; j<column; j++)\n      {\n    if(matrix[i][j]<0)matrix[i][j]=length_alph+matrix[i][j];\n \n      }\n}"("matrix"=w285, "length_alph"=w274, "column"=w283, "row"=w284) -> ("matrix"=w240:i32[][])
                      "обратная по модулю к матрице ключа" <- w240
                      n187 = call-poly <vilib>:"A x B.vi"("B"=w282, "A"=w240) -> ("A x B"=w276:T2)  [unwired: 1 out]
                      n188 = Matrix Size(0:w276) -> (1:w281:i32, 2:w280:i32)
                      n189 = formula code="int32 i =0;  int32 j=0;\nfor(  i=0; i<row; i++)\n{\n    for(  j=0; j<column; j++)\n      {\n     matrix[i][j]=mod(matrix[i][j],length_alph);\n      }\n}"("matrix"=w276, "length_alph"=w274, "column"=w280, "row"=w281) -> ("matrix"=→"Проверка":T2)
                      n190 = constructor class="Class1"() -> (reference out=w255:refnum<k24>, error out=w253:errorcluster)  [unwired: 3 in, 1 out]
                      n191 = global write "Global 1.vi" "tmp"(0 ("Numeric Control")) -> ()
                      n192 = Matrix Size(0:w240) -> (2:w256:i32)  [unwired: 1 out]
                      n193 = for {
                        N: "дл.исх.сообщ." -> [_]
                        tunnel: w256 -> [w341]
                        tunnel: w255 -> [w351]
                        tunnel: w253 -> [w349]
                        shift-right: [w347] -> w248
                        shift-left: "" -> [w348]
                        shift-right: [w339] -> w244
                        shift-left: _ -> [_]
                        shift-right: [w338] -> w243
                        shift-left: _ -> [_]
                        tunnel: w240 -> [w337]
                        tunnel: w238 -> [w336]
                        n194 = for {
                          N: w341 -> [_]
                          shift-right: [w366] -> w355
                          shift-left: "" -> [w369]
                          tunnel: w336 -> [w365]
                          n195 = global read "Global 1.vi" "tmp"() -> (w370:i32)
                          n196 = Index Array(array=w365, index=w370) -> (element=w364:i32)
                          n197 = Increment(x=w370) -> (x+1=w371:i32)
                          n198 = Number To Decimal String(number=w364) -> (decimal integer string=w368:string)  [unwired: 1 in]
                          n199 = global write "Global 1.vi" "tmp"(w371) -> ()
                          n200 = Concatenate Strings(w369, w368, " ") -> (w366:string)
                        }
                        n201 = Spreadsheet String To Array(delimiter (Tab)=" ", format string="", spreadsheet string=w355, array type (2D Dbl)=0) -> (array=w344:i32[][])
                        n202 = Matrix Size(0:w344) -> (2:w345:i32)  [unwired: 1 out]
                        n203 = Decrement(x=w345) -> (x-1=w346:i32)
                        n204 = invoke class="Class1" method="matrix_convert_1D"(reference=w351, error in=w349, "matrix"=w344, "column"=w346) -> (reference out=w339:refnum<k24>, error out=w338:errorcluster, "matrix_convert_1D"=w343:i32[])  [unwired: 1 in, 2 out]
                        n205 = call-poly <vilib>:"A x B.vi"("Matrix A"=w337, "Vector V'"=w343) -> ("V' x A"=w342:dbl[])  [unwired: 1 out]
                        n206 = for {
                          N: w341 -> [_]
                          shift-right: [w360] -> w340
                          shift-left: "" -> [w363]
                          tunnel: w342 -> [w358]
                          i -> [w359]
                          n207 = Index Array(array=w358, index=w359) -> (element=w357:dbl)
                          n208 = Number To Decimal String(number=w357) -> (decimal integer string=w362:string)  [unwired: 1 in]
                          n209 = Concatenate Strings(w363, w362, " ") -> (w360:string)
                        }
                        n210 = Concatenate Strings(w348, w340) -> (w347:string)
                      }
                      n211 = global read "Global 1.vi" "Вх. масс. алф."() -> (w270:string[][])
                      n212 = Matrix Size(0:w270) -> (2:w271:i32)  [unwired: 1 out]
                      n213 = Spreadsheet String To Array(delimiter (Tab)=" ", format string="", spreadsheet string=w248, array type (2D Dbl)=0) -> (array=w245:i32[][])
                      n214 = Matrix Size(0:w245) -> (2:w247:i32)  [unwired: 1 out]
                      n215 = Decrement(x=w247) -> (x-1=w246:i32)
                      n216 = invoke class="Class1" method="matrix_convert_1D"(reference=w244, error in=w243, "matrix"=w245, "column"=w246) -> (reference out=w242:refnum<k24>, error out=w241:errorcluster, "matrix_convert_1D"=w239:i32[])  [unwired: 1 in, 2 out]
                      n217 = Array Size(array=w239) -> (size(s)=w273:i32)
                      n218 = formula code="int32 i =0;\nfor(  i=0; i<size; i++)\n{\n     vector[i]=mod(vector[i],length_alph);\n}"("vector"=w239, "size"=w273, "length_alph"=w274) -> ("vector"=w272:i32[])
                      "Исходное сообщение" <- w272
                      n219 = call-poly <vilib>:"Array To Matrix.vi"("Real 1D Array"=w272) -> ("Real Matrix (Column Vector)"=w259:T2)
                      n220 = Transpose 2D Array(2D array=w259) -> (transposed array=w258:T2)
                      n221 = Matrix Size(0:w258) -> (1:w269:i32, 2:w268:i32)
                      n222 = invoke class="Class1" method="matrix_deshifr"(reference=w267, error in=w266, "str"=w270, "leng"=w271, "matrix"=w258, "row"=w269, "column"=w268) -> (reference out=w265:refnum<k24>, error out=w264:errorcluster, "matrix_deshifr"=w263:string[][])  [unwired: 1 in, 5 out]
                      n223 = Close Reference(reference=w265, error in (no error)=w264) -> ()  [unwired: 1 out]
                      n224 = Array To Spreadsheet String(delimiter (Tab)="", array=w263, 3:"" ("format string")) -> (spreadsheet string=→"Исходное сообщение":string)
                      n225 = Close Reference(reference=w242, error in (no error)=w241) -> ()  [unwired: 1 out]
                    }
                  }
                }
              }
            }
          }
        }
      }
    }
    frame #1 {
      n226 = Quit LabVIEW(quit? (T)=TRUE) -> ()
    }
  }
